vi "Multiread.vi"(0 "Keithley 2450":refnum<visa-resource-name>, 1 "Keithley Config":T1={"Source Compliance (A)"=0.1, "Min Voltage (V)"=0.0, "Max Voltage (V)"=5.0, "Source Mode"=0, "Number of Points"=50} {"Number of Points" min=2 step=1; "Source Mode" items=["Voltage", "Current"]; "Min Voltage (V)" min=0.1}, 5 "6510":refnum<visa-resource-name>, 7 "Number of Sensors":i16, 9 "2450 error in":errorcluster, 11 "6510 error in":errorcluster, 12 "t0 2":dbl) -> (4 "2450 Visa":refnum<visa-resource-name>, 6 "6510 Visa":refnum<visa-resource-name>, 8 "All Values Out":sgl[][][](array[numeric]), 10 "Resistance (ohm) Out":dbl[][](array[numeric]), 15 "Total Read Time":dbl)   [LabVIEW 2019, in "SMU.lvclass"]
uses:
  SMU.lvclass
  typeDefs/keithleySettings.ctl
  <instrlib>/Keithley DMM6500 DAQ6500 Series/Keithley DMM6500 DAQ6500 Series.lvlib
panel:
  out "6510Error Out":errorcluster
  out "2450 Error Out":errorcluster
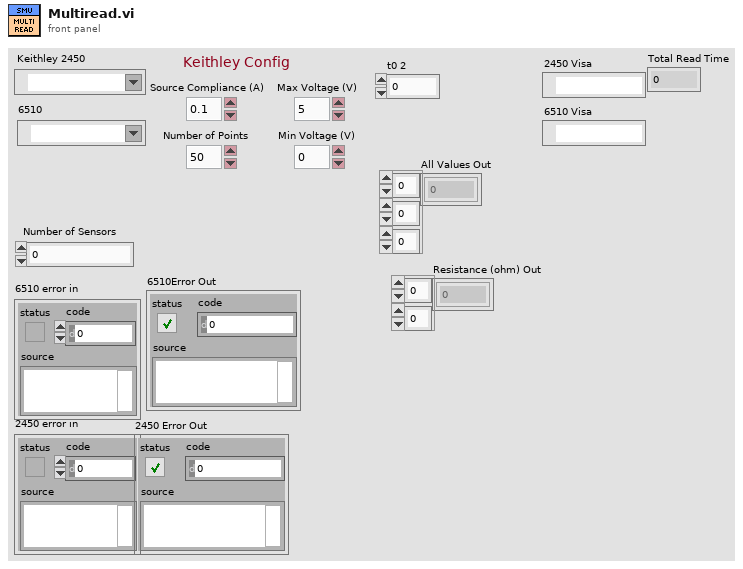
[diagram p1: front panel]
types:
  T1 = typedef "keithleySettings.ctl" = cluster{"Source Compliance (A)":dbl, "Min Voltage (V)":dbl, "Max Voltage (V)":dbl, "Source Mode":u16, "Number of Points":u32}
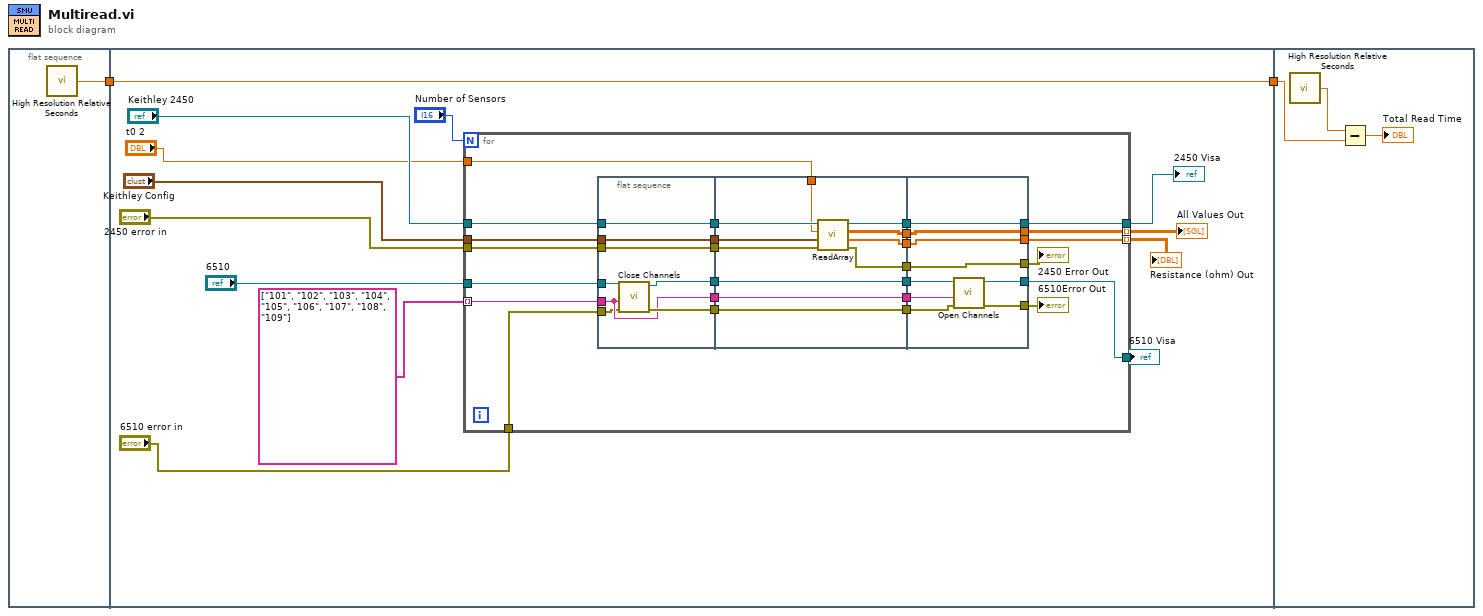
[diagram p0: block diagram]
diagram:
  n1 = flat-sequence {
    tunnel: [w3] -> w2
    tunnel: w2 -> [w4]
    tunnel: [w4] -> w1
    tunnel: w1 -> [w72]
    frame #0 {
      n2 = call <vilib>:"High Resolution Relative Seconds.vi"() -> ("relative seconds"=w3:dbl)
    }
    frame #1 {
      n3 = for {
        N: "Number of Sensors" -> [_]
        tunnel: "Keithley 2450" -> [w42]
        tunnel: "2450 error in" -> [w41]
        tunnel: "Keithley Config" -> [w40]
        tunnel: string[] ["101", "102", "103", "104", "105", "106", "107", "108", "109"] -> [w36] mode=indexing
        tunnel: "6510" -> [w35]
        tunnel: "6510 error in" -> [w22]
        tunnel: [w21] -> w7
        tunnel: [w20] -> w9 mode=indexing
        tunnel: [w19] -> w8 mode=indexing
        tunnel: [w18] -> w6
        tunnel: "t0 2" -> [w17]
        n4 = flat-sequence {
          tunnel: w40 -> [w48]
          tunnel: w41 -> [w49]
          tunnel: w42 -> [w50]
          tunnel: [w50] -> w39
          tunnel: [w49] -> w38
          tunnel: [w48] -> w37
          tunnel: w36 -> [w44]
          tunnel: w35 -> [w47]
          tunnel: [w46] -> w33
          tunnel: [w45] -> w32
          tunnel: [w44] -> w30
          tunnel: w22 -> [w43]
          tunnel: w39 -> [w61]
          tunnel: w38 -> [w60]
          tunnel: w37 -> [w59]
          tunnel: [w58] -> w34
          tunnel: w33 -> [w58]
          tunnel: w32 -> [w57]
          tunnel: [w57] -> w31
          tunnel: w30 -> [w56]
          tunnel: [w56] -> w29
          tunnel: [w55] -> w28
          tunnel: [w54] -> w27
          tunnel: [w53] -> w26
          tunnel: [w52] -> w25
          tunnel: w17 -> [w51]
          tunnel: w34 -> [w70]
          tunnel: w31 -> [w69]
          tunnel: w29 -> [w68]
          tunnel: [w67] -> w21
          tunnel: w28 -> [w67]
          tunnel: [w66] -> w20
          tunnel: w27 -> [w66]
          tunnel: [w65] -> w19
          tunnel: w26 -> [w65]
          tunnel: [w64] -> w24
          tunnel: w25 -> [w64]
          tunnel: [w63] -> w23
          tunnel: [w62] -> w18
          frame #0 {
            n5 = call <instrlib>:"Close Channels.vi"("error in (no error)"=w43, "Channel List(\"\")"=w44, "VISA resource name"=w47) -> ("error out"=w45:errorcluster, "VISA resource name out"=w46:refnum<visa-resource-name>)  [unwired: 7 in]
          }
          frame #1 {
            n6 = call "ReadArray.vi"("error in (no error)"=w60, "Keithley Config"=w59, "t0 2"=w51, "VISA resource name"=w61) -> ("error out"=w52:errorcluster, "Resistance (ohm)"=w53:dbl[], "appended array"=w54:sgl[][], "VISA resource name out"=w55:refnum<visa-resource-name>)  [unwired: 4 in]
          }
          frame #2 {
            n7 = call <instrlib>:"Open Channels.vi"("error in (no error)"=w69, "Channel List(\"\")"=w68, "VISA resource name"=w70) -> ("error out"=w63:errorcluster, "VISA resource name out"=w62:refnum<visa-resource-name>)  [unwired: 7 in]
          }
        }
        "2450 Error Out" <- w24
        "6510Error Out" <- w23
      }
      "All Values Out" <- w9
      "Resistance (ohm) Out" <- w8
      "2450 Visa" <- w7
      "6510 Visa" <- w6
    }
    frame #2 {
      n8 = call <vilib>:"High Resolution Relative Seconds.vi"() -> ("relative seconds"=w73:dbl)
      n9 = Subtract(x=w73, y=w72) -> (x-y=→"Total Read Time":dbl)
    }
  }
